vi "GT Crd Status.vi"(6 "fifo":i16, 7 "pSegment":i32, 8 "error in (no error)":errorcluster caption="错误输入（无错误）", 9 "pRun":i16, 10 "crd":i16, 11 "cardNum":i16) -> (0 "error out":errorcluster caption="错误输出", 1 "pRun out":i16, 3 "function return":i16, 5 "pSegment out":i32)   [LabVIEW 2014, in "gts.lvlib"]
doc: "GT_API GT_CrdStatus(short cardNum,short crd,short *pRun,long *pSegment,short fifo=0);"
uses:
  gts.lvlib
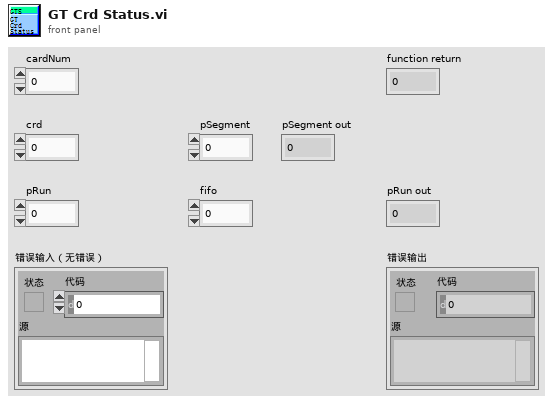
[diagram p1: front panel]
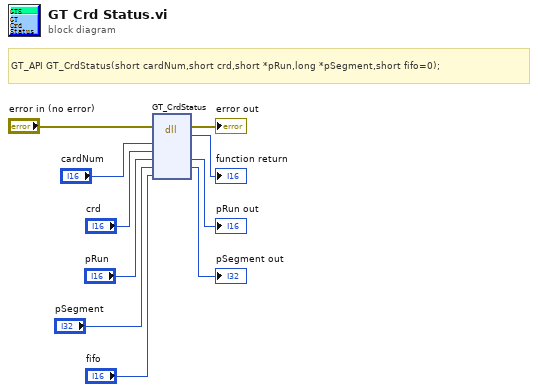
[diagram p0: block diagram]
diagram:
  # "GT_API GT_CrdStatus(short cardNum,short crd,short *pRun,long *pSegment,short fifo=0);"
  n1 = dll-call lib="PTH2habs D固高科技资料GTS控制卡GTS卡18年上半年资料dllVC32bit\nmulti_cardgts.*" fn="GT_CrdStatus"(error in="error in (no error)", "cardNum"="cardNum", "crd"="crd", "pRun"="pRun", "pSegment"="pSegment", "fifo"="fifo") -> (error out=→"error out":errorcluster, →"function return":i16, "pRun"=→"pRun out":i16, "pSegment"=→"pSegment out":i32)  [unwired: 5 in, 1 out]
